vi "Read File.vi"(8 "Error In":errorcluster) -> (0 "Error Out":errorcluster, 3 "Zone Set Up":cluster{"Zone Selector":string, "Timing":dbl}[](array[cluster]))   [LabVIEW 2024]
uses:
  <vilib>/Utility/file.llb/Read Delimited Spreadsheet (string).vi
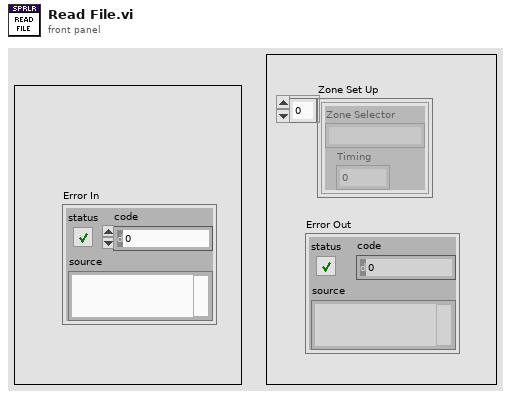
[diagram p1: front panel]
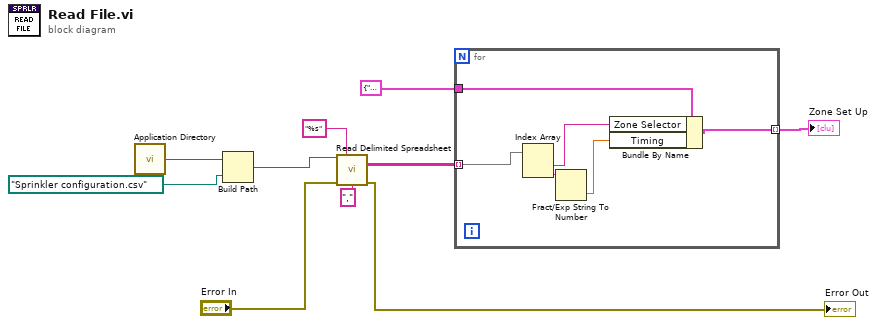
[diagram p0: block diagram]
diagram:
  n1 = call <vilib>:"Application Directory.vi"() -> ("Application Directory"=w3:path)
  n2 = Build Path(base path=w3, name or relative path=path "Sprinkler configuration.csv" ("Path")) -> (appended path=w5:path)
  n3 = call-poly <vilib>:"Read Delimited Spreadsheet.vi"("file path (dialog if empty)"=w5, "format (%s)"="%s", "error in (no error)"="Error In", "delimiter (\\t)"="," ("delimiter (\\t)")) -> ("all rows"=w9:string[][], "error out"=→"Error Out":errorcluster)  [unwired: 6 in, 4 out]
  n4 = for {
    tunnel: cluster{"Zone Selector":string, "Timing":dbl} {"Zone Selector"="", "Timing"=0.0} ("Zone Selector") -> [w16]
    tunnel: w9 -> [w15] mode=indexing
    tunnel: [w11] -> w10 mode=indexing
    n5 = Index Array(array=w15) -> (element #1=w14:string, element #2=w13:string)  [unwired: 2 in]
    n6 = Fract/Exp String To Number(string=w13) -> (number=w12:dbl)  [unwired: 3 in, 1 out]
    n7 = Bundle By Name(cluster=w16, "Zone Selector"=w14, "Timing"=w12) -> (w11:cluster{"Zone Selector":string, "Timing":dbl})
  }
  "Zone Set Up" <- w10
